vi "one second acquisition loop.vi"(8 "error in (no error)":errorcluster, 11 "DAQCascade512II":refnum<class "DAQCascade512II.lvclass">) -> (0 "error out":errorcluster, 3 "DAQCascade512II out":refnum<class "DAQCascade512II.lvclass">)   [LabVIEW 2012, in "DAQCascade512II.lvclass"]
uses:
  DAQCascade512II.lvclass
  DAQCascade512II.lvclass/DAQCascade512II.ctl
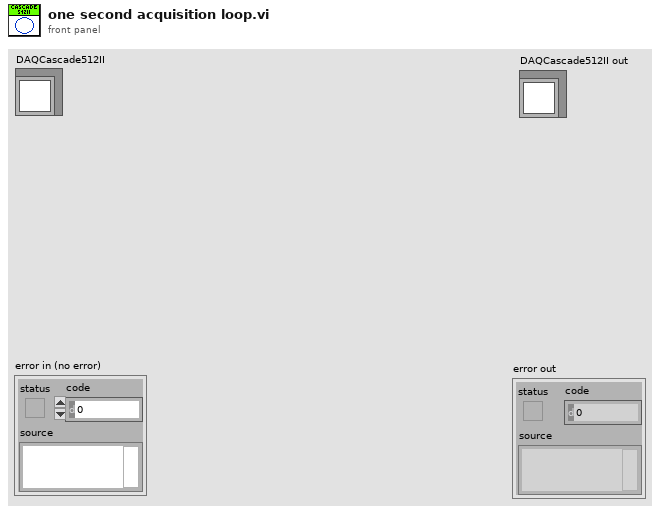
[diagram p1: front panel]
types:
  T1 = cluster{"Rows Per Strip":i32, "Photometric":i32, "Compression Type":i32}
  T2 = typedef "DAQCascade512II.lvclass/File Path.ctl" = path
  T3 = typedef "IMAQ Image.ctl" = refnum<image>
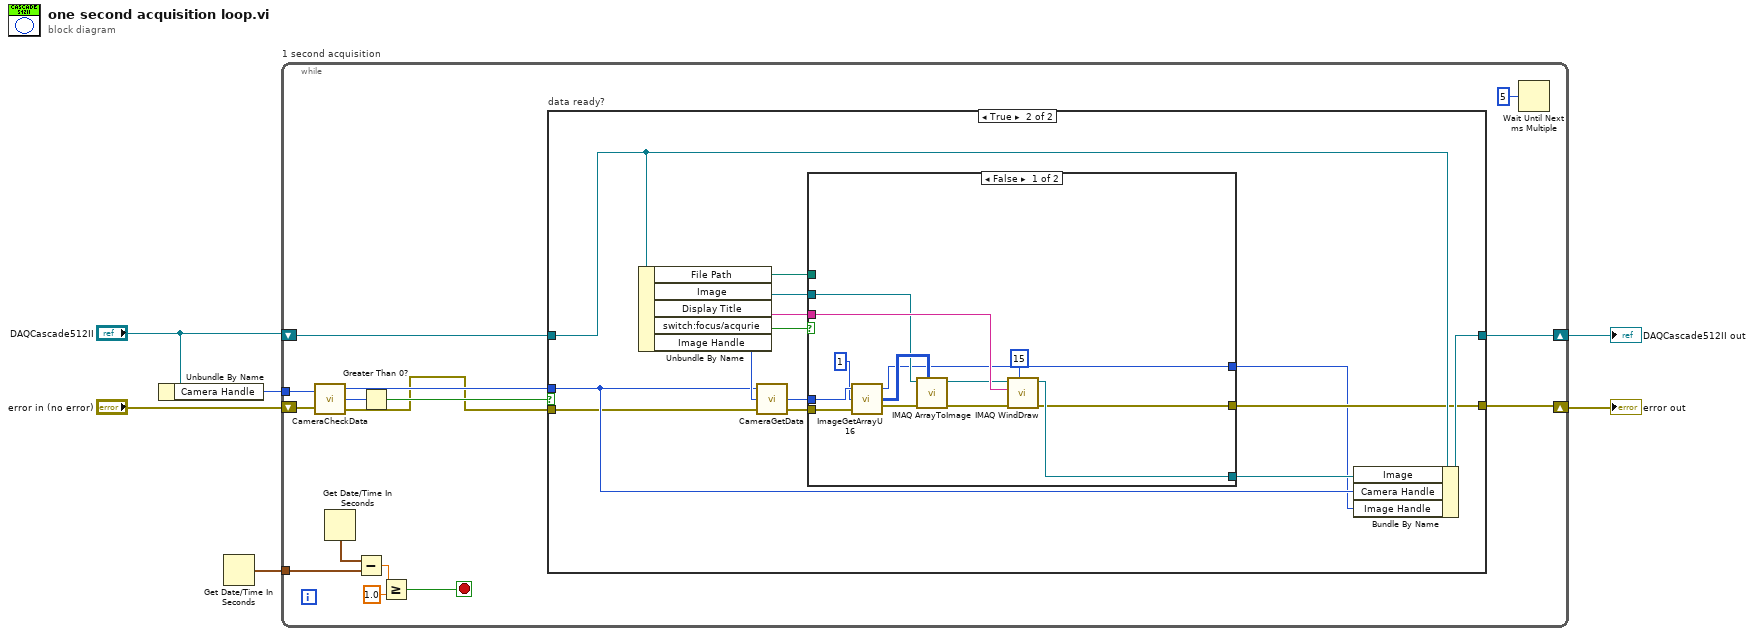
[diagram p0: block diagram]
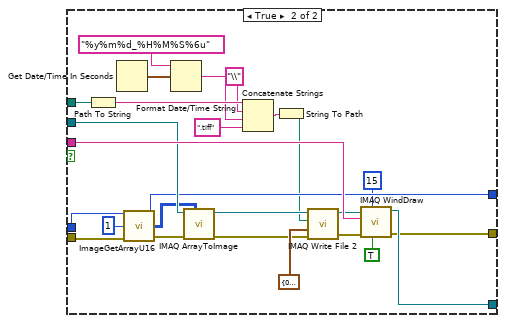
[diagram p3: hidden frame]
diagram:
  n1 = Unbundle By Name("DAQCascade512II") -> ("Camera Handle"=w2:u32)
  n2 = Get Date/Time In Seconds() -> (seconds since 1Jan1904=w1:timestamp)
  n3 = while "1 second acquisition" {
    tunnel: w2 -> [w21]
    shift-right: [w13] -> w4
    shift-left: "error in (no error)" -> [w18]
    shift-right: [w16] -> w5
    shift-left: "DAQCascade512II" -> [w7]
    tunnel: w1 -> [w11]
    stop <- w14 stop-if-true
    n4 = call <userlib>:"CameraCheckData.vi"("Camera Handle"=w21, "error in"=w18) -> ("Camera Handle"=w17:u32, "Number Of Frames Available"=w20:i32, "error out"=w8:errorcluster)
    n5 = Get Date/Time In Seconds() -> (seconds since 1Jan1904=w12:timestamp)
    n6 = Subtract(x=w12, y=w11) -> (x-y=w10:dbl)
    n7 = Greater Than 0?(x=w20) -> (x > 0?=w19:bool)
    n8 = Greater Or Equal?(x=w10, y=1.0) -> (x >= y?=w14:bool)
    n9 = case "data ready?" shown="True" w19 {
      tunnel: w17 -> [_ w29]
      tunnel: w7 -> [w23 w37]
      tunnel: w8 -> [w22 w28]
      tunnel: [w23 w36] -> w16
      tunnel: [w22 w35] -> w13
      frame False {
      }
      frame True {
        n10 = Unbundle By Name(w37) -> ("File Path"=w24:T2, "Image"=w31:T3, "Display Title"=w32:string, "switch:focus/acqurie"=w34:bool, "Image Handle"=w30:u32)
        n11 = call <userlib>:"CameraGetData.vi"("error in"=w28, "Data Handle"=w30, "Camera Handle"=w29) -> ("error out"=w27:errorcluster, "Data Handle"=w26:u32)  [unwired: 1 out]
        n12 = case shown="False" w34 {
          tunnel: w27 -> [w46 w76]
          tunnel: w32 -> [w50 w75]
          tunnel: [w47 w70] -> w35
          tunnel: [w48 w73] -> w33
          tunnel: w31 -> [w40 w74]
          tunnel: w26 -> [w45 w72]
          tunnel: [w38 w71] -> w25
          tunnel: w24 -> [_ w55]
          frame False {
            n13 = call <userlib>:"ImageGetArrayU16.vi"("error in"=w46, "Z position"=u32 1, "Image Handle"=w45) -> ("error out"=w42:errorcluster, "Array uint 16"=w43:u16[][], "Image Handle"=w38:u32)
            n14 = call "IMAQ ArrayToImage"("Image Pixels (U16)"=w43, "error in (no error)"=w42, "Image"=w40) -> ("error out"=w41:errorcluster, "Image Out"=w39:T3)  [unwired: 7 in]
            n15 = call "IMAQ WindDraw"("Window Number (0...15)"=15, "error in (no error)"=w41, "Title"=w50, "Image"=w39) -> ("error out"=w47:errorcluster, "Image Out (duplicate)"=w48:T3)  [unwired: 6 in]
          }
          frame True {
            n16 = Path To String(path=w55) -> (string=w61:string)
            n17 = Get Date/Time In Seconds() -> (seconds since 1Jan1904=w62:timestamp)
            n18 = call <userlib>:"ImageGetArrayU16.vi"("error in"=w76, "Z position"=u32 1, "Image Handle"=w72) -> ("error out"=w67:errorcluster, "Array uint 16"=w68:u16[][], "Image Handle"=w71:u32)
            n19 = Format Date/Time String(time format string (%c)="%y%m%d_%H%M%S%6u", seconds (now)=w62) -> (date/time string=w59:string)  [unwired: 1 in]
            n20 = call "IMAQ ArrayToImage"("Image Pixels (U16)"=w68, "error in (no error)"=w67, "Image"=w74) -> ("error out"=w56:errorcluster, "Image Out"=w54:T3)  [unwired: 7 in]
            n21 = Concatenate Strings(w61, "\\" ("string"), w59, ".tiff" ("string")) -> (w57:string)
            n22 = String To Path(string=w57) -> (path=w53:path)
            n23 = call-poly "IMAQ Write File 2"("error in (no error)"=w56, "TIFF Options"=T1 {"Rows Per Strip"=0, "Photometric"=1, "Compression Type"=0}, "File Path"=w53, "Image"=w54) -> ("error out"=w52:errorcluster, "Image Out (duplicate)"=w51:T3)  [unwired: 6 in]
            n24 = call "IMAQ WindDraw"("Resize to Image Size? (Y)"=TRUE, "Window Number (0...15)"=15, "error in (no error)"=w52, "Title"=w75, "Image"=w51) -> ("error out"=w70:errorcluster, "Image Out (duplicate)"=w73:T3)  [unwired: 5 in]
          }
        }
        n25 = Bundle By Name(cluster=w37, "Image"=w33, "Camera Handle"=w29, "Image Handle"=w25) -> (w36:refnum<class "DAQCascade512II.lvclass">)
      }
    }
    n26 = Wait Until Next ms Multiple(millisecond multiple=u32 5) -> ()  [unwired: 1 out]
  }
  "error out" <- w4
  "DAQCascade512II out" <- w5
